vi "Msg.vi"(7 "LVCAM in":refnum<class "LVCAM.lvclass">, 11 "LVCAM Destroy Self Msg in":refnum<class "LVCAM Destroy Self Msg.lvclass">) -> (0 "error out":errorcluster, 2 "Destroyed Self?":bool, 5 "LVCAM out":refnum<class "LVCAM.lvclass">)   [LabVIEW 2021, in "LVCAM Destroy Self.lvlib" / "LVCAM Destroy Self Msg.lvclass"]
uses:
  LVCAM Destroy Self Msg.lvclass
  LVCAM/LVCAM/LVCAM.lvclass
  LVCAM Destroy Self/LVCAM Destroy Self.lvclass
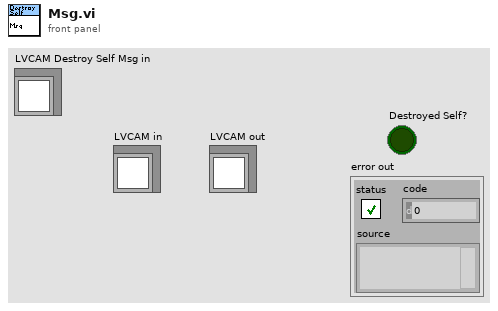
[diagram p1: front panel]
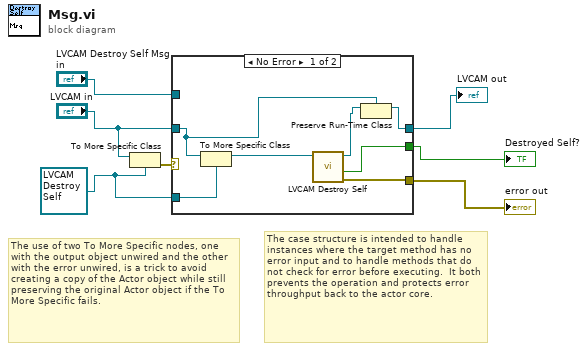
[diagram p0: block diagram]
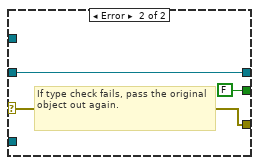
[diagram p2: hidden frame]
diagram:
  w1 = refnum<class "LVCAM Destroy Self.lvclass"> refnum ("Destroy.lvlib:Destroy.lvclass")
  # "The use of two To More Specific nodes, one with the output object unwired and the other with the error unwired, is a trick to avoid creating a copy of the Actor object while still preserving the original Actor object if the To More Specific fails."
  # "The case structure is intended to handle instances where the target method has no error input and to handle methods that do not check for error before executing.  It both prevents the operation and protects error throughput back to the actor core."
  n1 = To More Specific Class(target class=w1, reference="LVCAM in") -> (error out=w7:errorcluster)  [unwired: 1 in, 1 out]
  n2 = case shown="No Error" w7 {
    selector: w7 -> [_ w17]
    tunnel: [w14 w17] -> w6
    tunnel: [w9 w16] -> w4
    tunnel: "LVCAM in" -> [w10 w16]
    tunnel: "LVCAM Destroy Self Msg in" -> [_ _]
    tunnel: [w8 FALSE ("Destroyed Self?")] -> w2
    tunnel: w1 -> [w12 _]
    frame No Error {
      n3 = To More Specific Class(target class=w12, reference=w10) -> (specific class reference=w13:refnum<class "LVCAM Destroy Self.lvclass">)  [unwired: 1 in, 1 out]
      n4 = call-dynamic "LVCAM Destroy Self.vi"("LVCAM Destroy Self in"=w13) -> ("error out"=w14:errorcluster, "Destroyed Self?"=w8:bool, "LVCAM Destroy Self out"=w11:refnum<class "LVCAM Destroy Self.lvclass">)  [unwired: 8 in]
      n5 = Preserve Run-Time Class(object in=w11, 2:w10) -> (object out=w9:refnum<class "LVCAM.lvclass">)  [unwired: 1 in, 1 out]
    }
    frame Error {
      # "If type check fails, pass the original object out again."
    }
  }
  "error out" <- w6
  "Destroyed Self?" <- w2
  "LVCAM out" <- w4
